vi "T-sql 替换参数.vi"(6 "替换项":cluster{"被替换":string, "替换为":string}[](array[cluster]), 8 "错误输入":errorcluster, 11 "T-sql 模板":string) -> (0 "错误输出":errorcluster, 3 "T-sql":string)   [LabVIEW 2017]
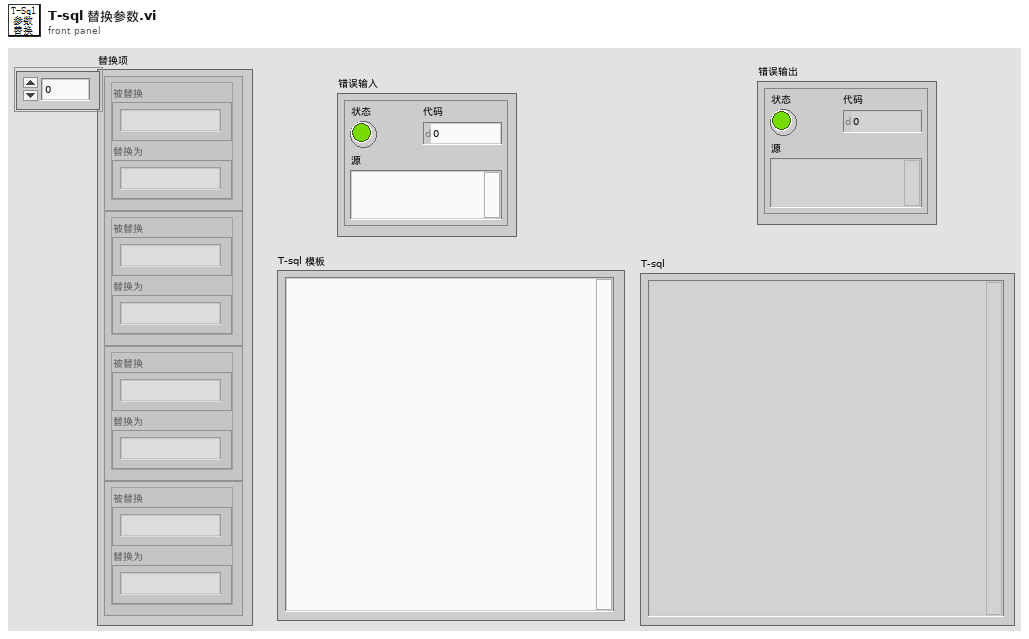
[diagram p1: front panel]
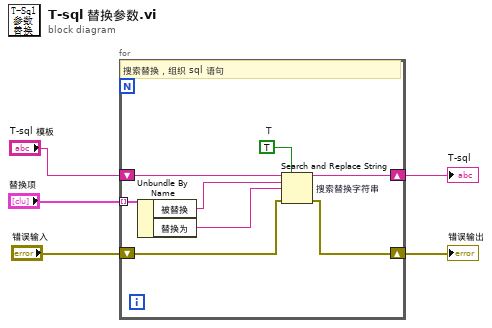
[diagram p0: block diagram]
diagram:
  n1 = for {
    shift-right: [w6] -> w3
    shift-left: "T-sql 模板" -> [w12]
    tunnel: "替换项" -> [w11] mode=indexing
    shift-right: [w7] -> w4
    shift-left: "错误输入" -> [w8]
    w13 = TRUE  # T
    # "搜索替换，组织 sql 语句"
    n2 = Unbundle By Name(w11) -> ("被替换"=w10:string, "替换为"=w9:string)
    n3 = Search and Replace String "搜索替换字符串"(replace all?=w13, input string=w12, search string=w10, replace string=w9, error in=w8) -> (result string=w6:string, error out=w7:errorcluster)  [unwired: 3 in, 2 out]
  }
  "错误输出" <- w4
  "T-sql" <- w3
